vi "Error Q v1_0_1.vi"(0 "Queue name":string="Error", 2 "rendezvous":T1, 3 "error in":errorcluster, 4 "Error Log File":path) -> (10 "error out":errorcluster)   [LabVIEW 2015]
doc: "Error Q v1_0_0.vi\n\nTest Error Control:\n\nProcesses errors and logs them for the Test application.\nthis vi processes any errors that get sent to it. It will build a text file at the location of the file path you provide. It must be either started before your statemachine if ran in the same block diagram. (note in this case it must be ran indepedently from the rest of the state machine. if you wire up the error out indicator it will stop the state machine from running.) The other option is to launch it through vi server or system executive.vi. \n\n\nafter it is started --> send the following command to the Error queue. \"open?True\" or \"open?False\". open tells this vi to put an open statement on the error file. if True is passed to it it will append new entries to the existing file. False tells it to make a new file and delete any existing file. \n\nAt the end of your program --> send the followiing command to the Error queue... \"close\".\nthis will place a close statement in the error file and stop this vi.\n\n\n\nDeveloped by:\n J. Daren Suntych\nNational Analytics 2002\n970-397-0764"
panel:
  in  "Tree":string(tree)
  # "<-  path, including name, for the log file."
  # "<-  rendevouz used to coordinate activities between\n     this VI and the application."
  # "To Avoid creating duplicate Error codes.  Use Ranges of 5000 - 9999 for custom e\ncode development"
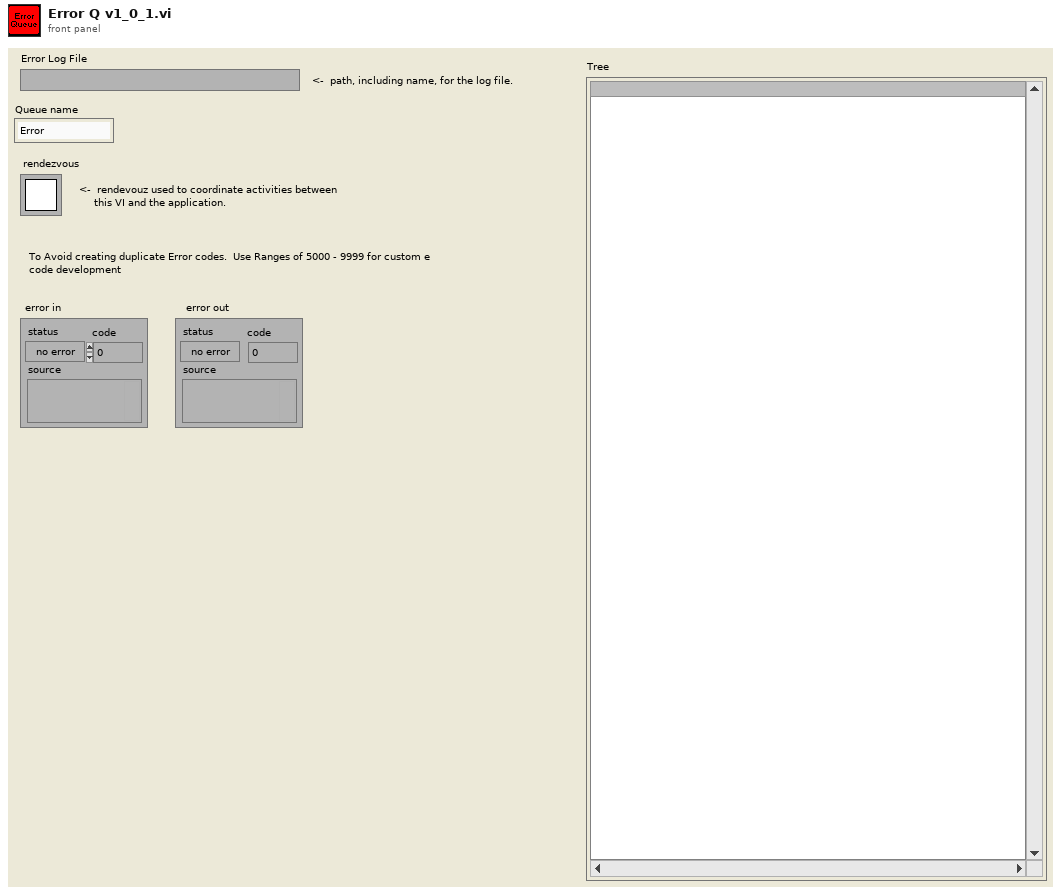
[diagram p1: front panel]
types:
  T1 = typedef "Rendezvous RefNum" = refnum<k1>
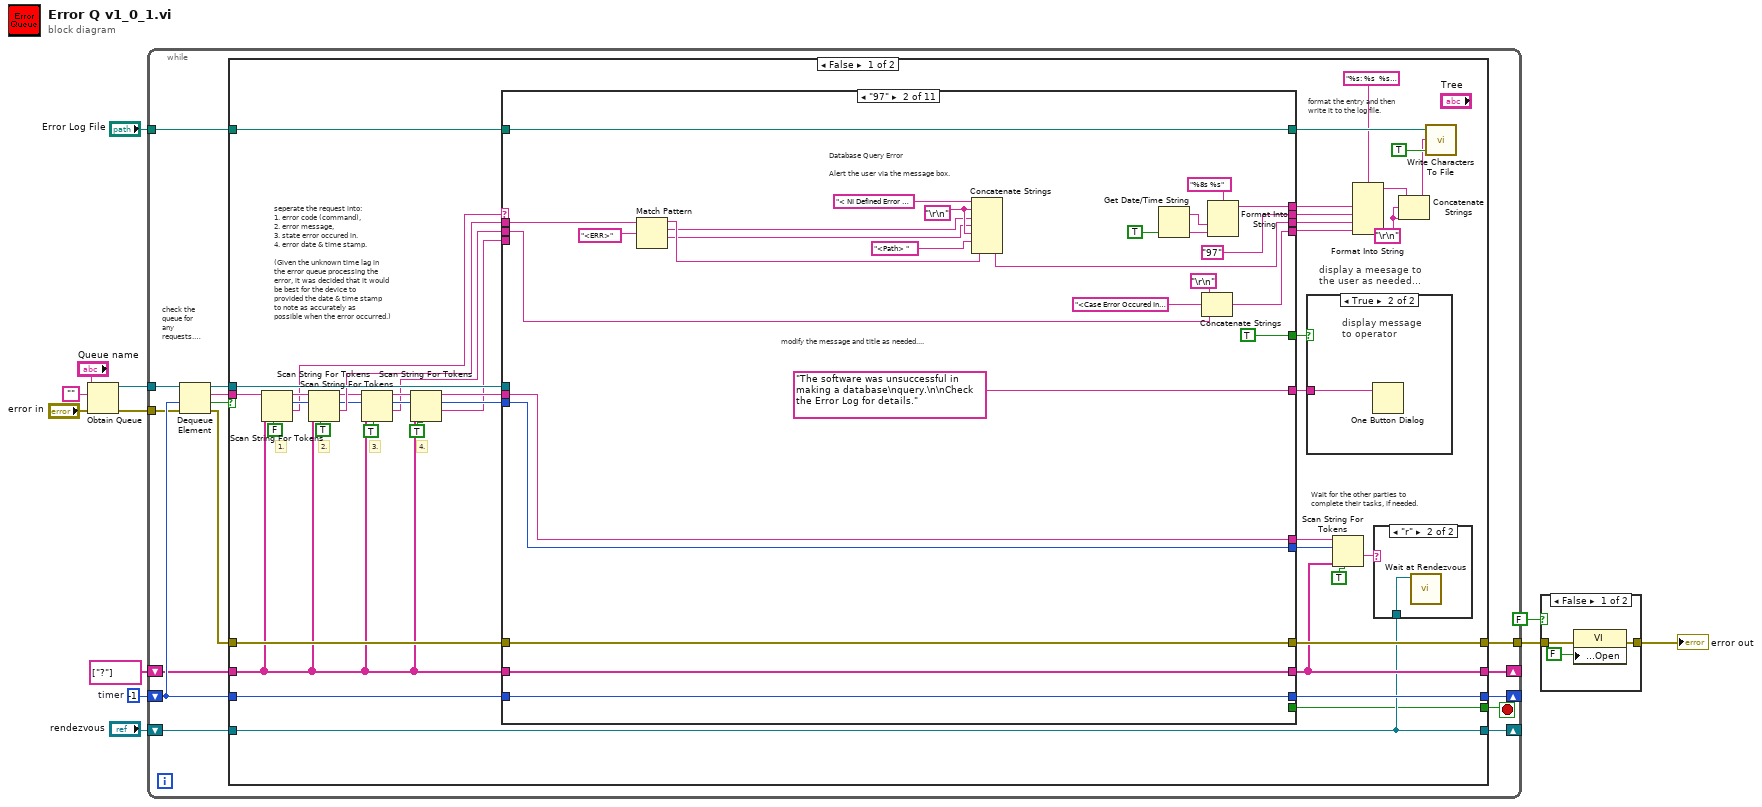
[diagram p0: block diagram]
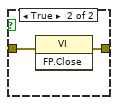
[diagram p2: hidden frame]
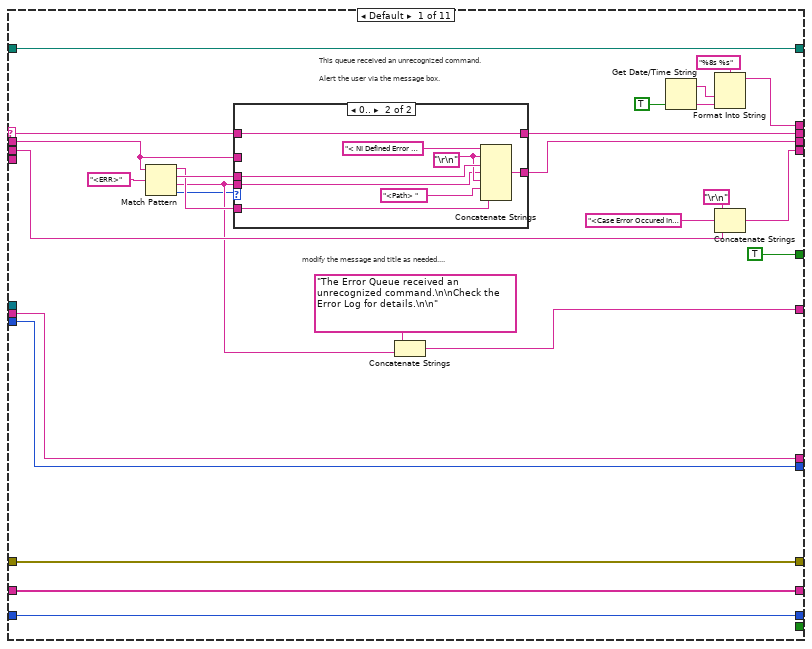
[diagram p5: hidden frame]
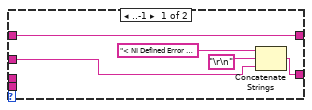
[diagram p6: hidden frame]
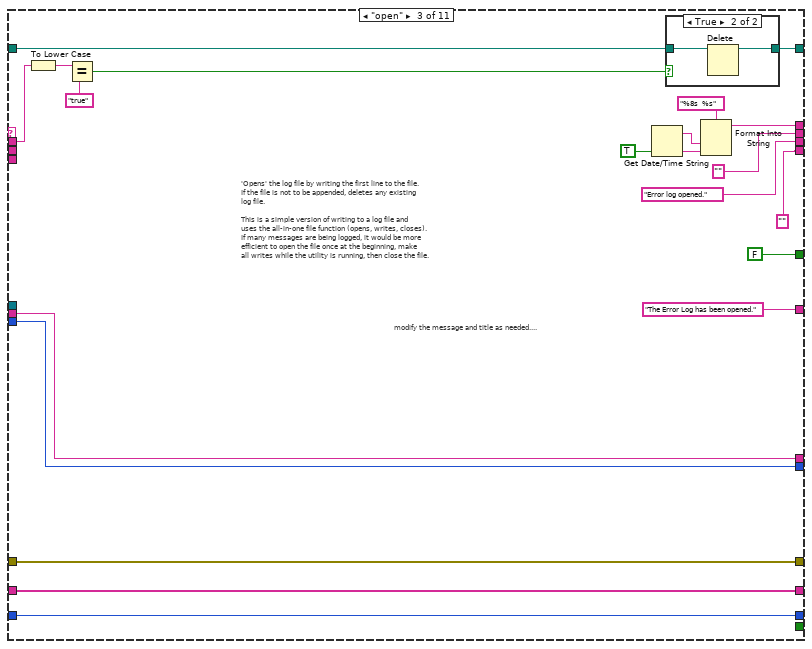
[diagram p7: hidden frame]
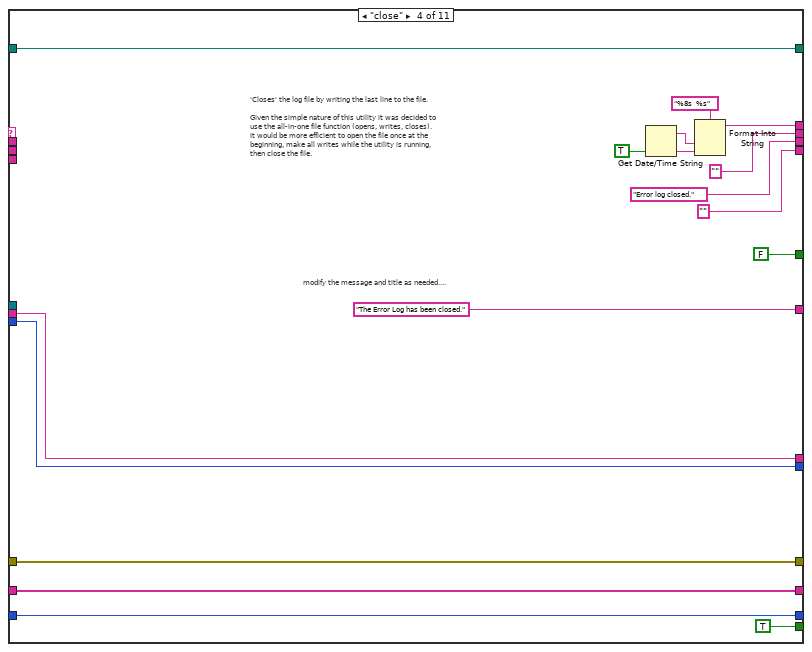
[diagram p9: hidden frame]
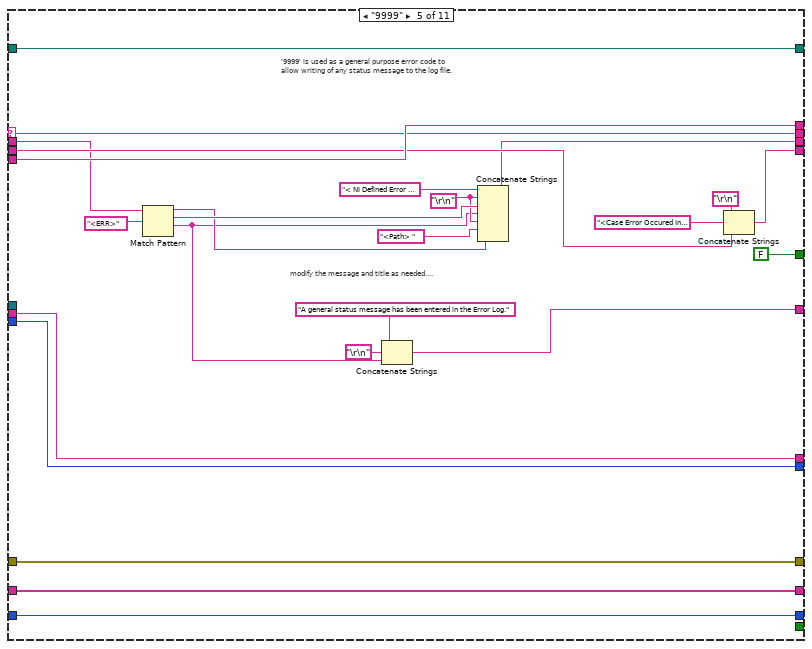
[diagram p10: hidden frame]
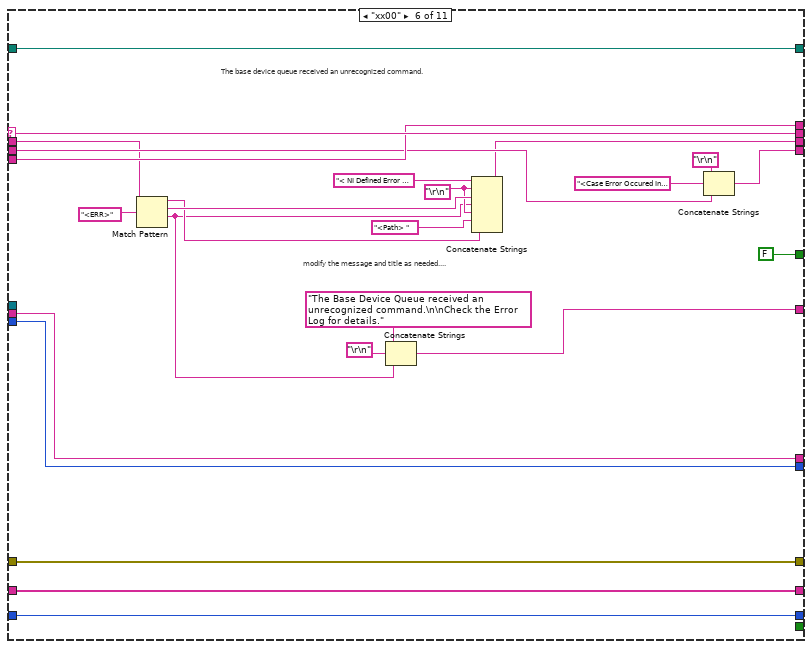
[diagram p11: hidden frame]
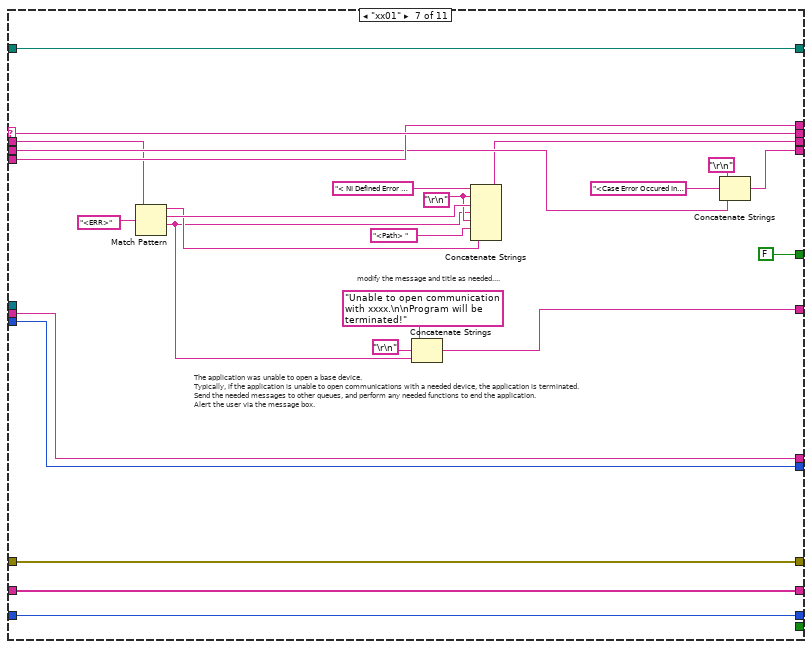
[diagram p12: hidden frame]
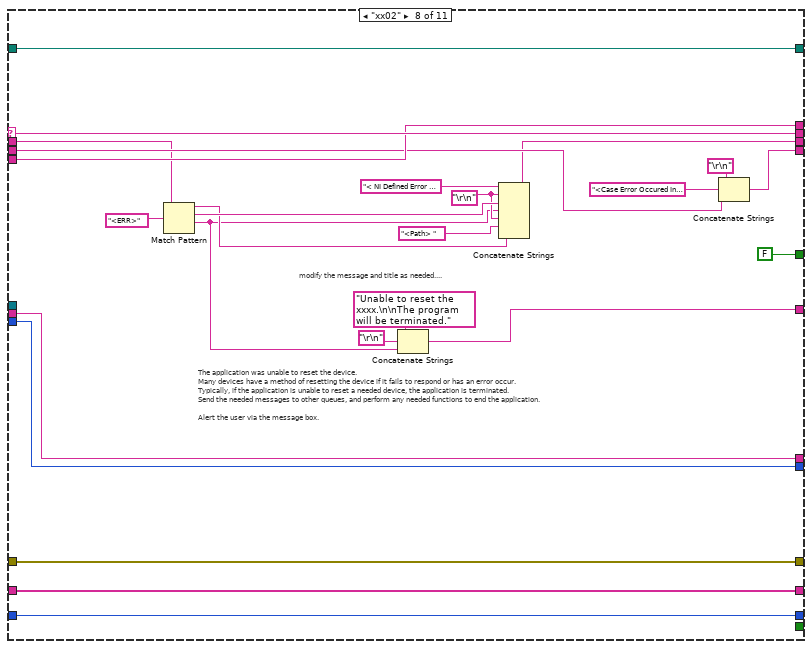
[diagram p13: hidden frame]
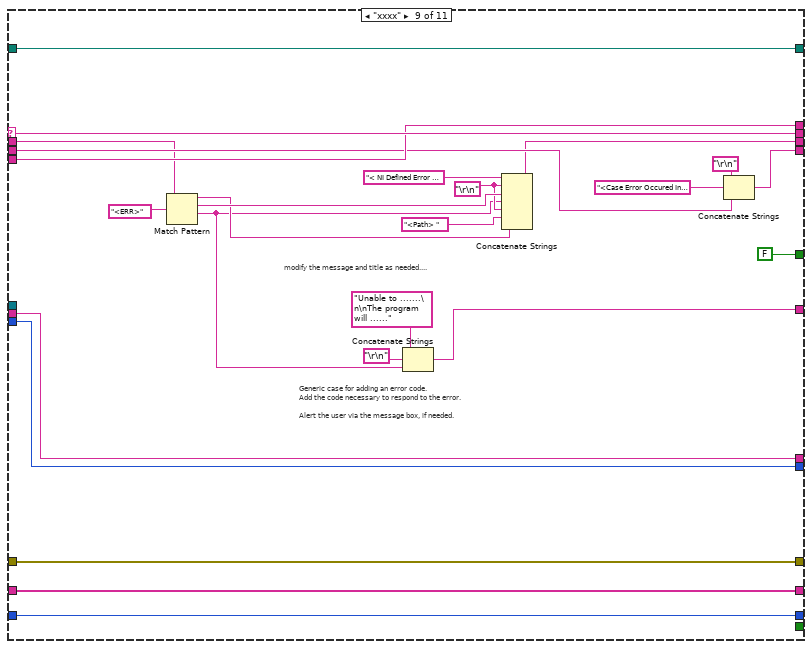
[diagram p14: hidden frame]
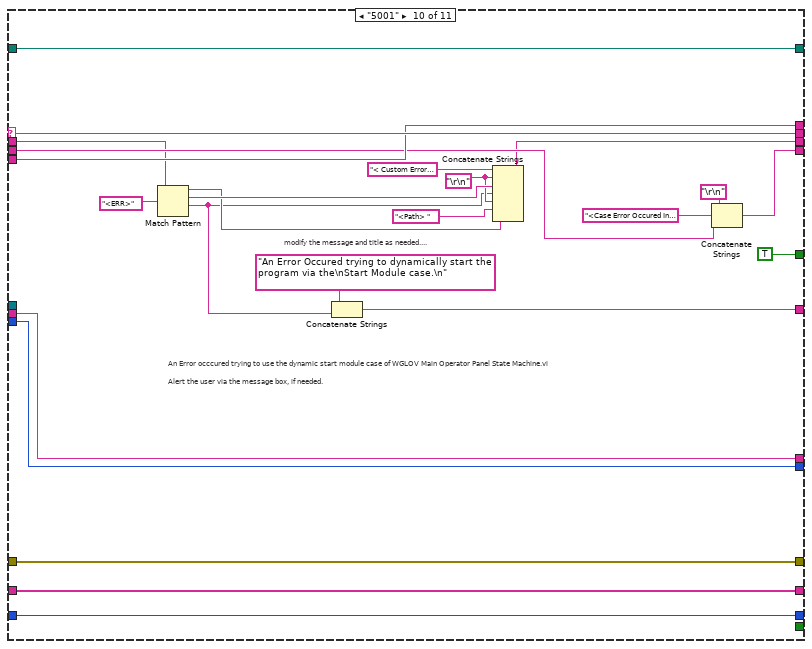
[diagram p15: hidden frame]
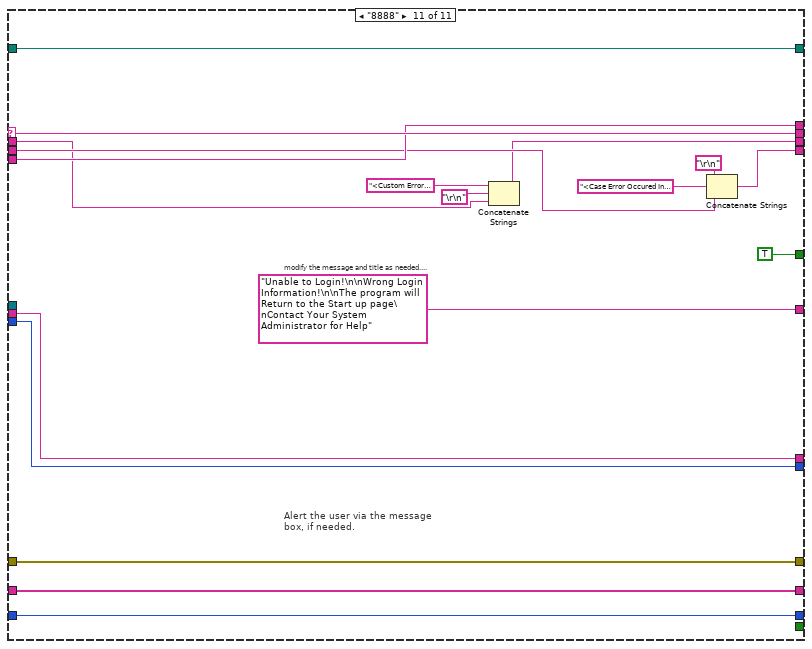
[diagram p16: hidden frame]
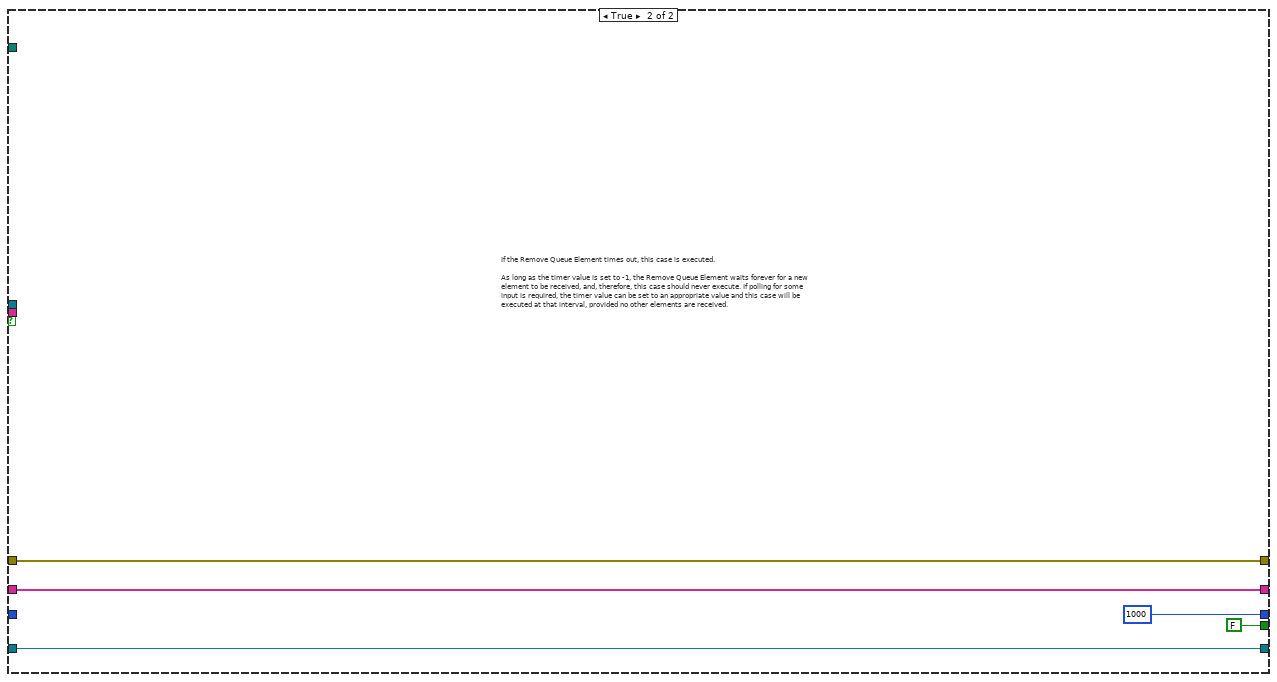
[diagram p17: hidden frame]
diagram:
  w12 = -1  # timer
  n1 = Obtain Queue(name (unnamed)="Queue name", element data type="", error in (no error)="error in") -> (queue out=w7:refnum<queue>, error out=w6:errorcluster)  [unwired: 2 in, 1 out]
  n2 = while {
    shift-left: "rendezvous" -> [w17]
    shift-right: [w16] -> _
    tunnel: "Error Log File" -> [w18]
    shift-left: string[] ["?"] ("Tokens") -> [w21]
    shift-right: [w20] -> _
    tunnel: w7 -> [w26]
    shift-left: w12 -> [w27]
    shift-right: [w22] -> _
    tunnel: [w19] -> w2
    tunnel: w6 -> [w13]
    stop <- w14 stop-if-true
    # "check the \nqueue for\nany \nrequests....."
    n3 = Dequeue Element(queue=w26, timeout in ms (-1)=w27, error in (no error)=w13) -> (queue out=w25:refnum<queue>, element=w24:string, timed out?=w23:bool, error out=w15:errorcluster)
    n4 = case shown="False" w23 {
      tunnel: [w64 w352] -> w19
      tunnel: w27 -> [w70 _]
      tunnel: w25 -> [w69 _]
      tunnel: w24 -> [w66 _]
      tunnel: w15 -> [w68 w352]
      tunnel: [w65 1000 ("timer")] -> w22
      tunnel: w21 -> [w28 w351]
      tunnel: [w48 w351] -> w20
      tunnel: w18 -> [w62 _]
      tunnel: w17 -> [w43 w350]
      tunnel: [w43 w350] -> w16
      tunnel: [w40 FALSE] -> w14
      frame False {
        w30 = "\r\n"
        # "3."
        # "4."
        # "2."
        # "1."
        # "format the entry and then\nwrite it to the log file."
        # "display a meesage to\nthe user as needed..."
        # "seperate the request into:\n1. error code (command),\n2. error message,\n3. state error occured in.\n4. error date & time stamp.\n\n(Given the unknown time lag in\nthe error queue processing the\nerror, it was decided that it would\nbe best for the device to\nprovided the date & time stamp\nto note as accurately as \npossible when the error occurred.)"
        # "Wait for the other parties to\ncomplete their tasks, if needed."
        n5 = Scan String For Tokens(4:FALSE ("use cached delim/oper data? (F)"), 6:w28, 9:w66) -> (1:w41:string, 2:w55:i32, 3:w54:string)  [unwired: 1 in, 3 out]
        n6 = Scan String For Tokens(4:TRUE ("use cached delim/oper data? (F)"), 6:w28, 8:w55, 9:w54) -> (1:w42:string, 2:w37:i32, 3:w39:string)  [unwired: 3 out]
        n7 = Scan String For Tokens(4:TRUE ("use cached delim/oper data? (F)"), 6:w28, 8:w37, 9:w39) -> (1:w35:string, 2:w36:i32, 3:w38:string)  [unwired: 3 out]
        n8 = Scan String For Tokens(4:TRUE ("use cached delim/oper data? (F)"), 6:w28, 8:w36, 9:w38) -> (1:w51:string, 2:w52:i32, 3:w53:string)  [unwired: 3 out]
        n9 = case shown="\"97\"" w41 {
          selector: w41 -> [w76 _ _ _ w199 w227 w253 w277 w302 w326 w344]
          tunnel: [w97 w137 w158 w178 w203 w229 w254 w279 w304 w328 w346] -> w64
          tunnel: w68 -> [w97 w137 w158 w178 w203 w229 w254 w279 w304 w328 w346]
          tunnel: w70 -> [w98 w138 w159 w179 w204 w230 w255 w280 w305 w329 w347]
          tunnel: w69 -> [_ _ _ _ _ _ _ _ _ _ _]
          tunnel: w28 -> [w99 w139 w160 w180 w205 w225 w251 w275 w300 w324 w342]
          tunnel: w52 -> [w89 w129 w145 w166 w197 w222 w248 w272 w297 w321 w339]
          tunnel: [w98 w138 w159 w179 w204 w230 w255 w280 w305 w329 w347] -> w65
          tunnel: [w99 w139 w160 w180 w205 w225 w251 w275 w300 w324 w342] -> w48
          tunnel: w53 -> [w85 w122 w146 w167 w198 w223 w249 w273 w298 w322 w340]
          tunnel: [w91 w131 w157 w177 w202 w228 w247 w278 w303 w327 w345] -> w61
          tunnel: w62 -> [w91 w131 w156 w177 w202 w228 w247 w278 w303 w327 w345]
          tunnel: [w92 w132 w151 w172 w200 w226 w252 w276 w301 w325 w343] -> w60
          tunnel: [w75 "97" "" "" w199 w227 w253 w277 w302 w326 w344] -> w59
          tunnel: [w77 w113 "Error log opened." "Error log closed." w185 w210 w235 w260 w285 w308 w332] -> w58
          tunnel: w42 -> [w73 w114 w144 _ w186 w211 w236 w262 w286 w307 w331]
          tunnel: w51 -> [_ _ _ _ w200 w226 w252 w276 w301 w325 w343]
          tunnel: [w87 "The software was unsuccessful in making a database\nquery.\n\nCheck the Error Log for details." "The Error Log has been opened." "The Error Log has been closed." w182 w207 w232 w257 w281 w320 "Unable to Login!\n\nWrong Login Information!\n\nThe program will Return to the Start up page\nContact Your System Administrator for Help"] -> w50
          tunnel: [TRUE TRUE FALSE FALSE FALSE FALSE FALSE FALSE FALSE TRUE TRUE] -> w49
          tunnel: [w85 w122 w146 w167 w198 w223 w249 w273 w298 w322 w340] -> w45
          tunnel: [w89 w129 w145 w166 w197 w222 w248 w272 w297 w321 w339] -> w44
          tunnel: [_ _ _ TRUE _ _ _ _ _ _ _] -> w40
          tunnel: w35 -> [w82 w123 _ _ w193 w218 w243 w268 w293 w315 w335]
          tunnel: [w86 w124 "" "" w194 w219 w244 w269 w294 w316 w336] -> w33
          frame Default {
            # "modify the message and title as needed...."
            # "This queue received an unrecognized command.\n\nAlert the user via the message box."
            n10 = Match Pattern(string=w73, regular expression="<ERR>") -> (before substring=w79:string, match substring=w80:string, after substring=w78:string, offset past match=w74:i32)  [unwired: 1 out]
            n11 = case shown="0.." w74 {
              tunnel: w80 -> [_ w111]
              tunnel: w79 -> [_ w108]
              tunnel: w78 -> [_ w107]
              tunnel: [w103 w106] -> w77
              tunnel: w76 -> [w102 w105]
              tunnel: [w102 w105] -> w75
              tunnel: w73 -> [w101 _]
              frame ..-1 {
                n12 = Concatenate Strings("< NI Defined Error > ", "\r\n", w101) -> (w103:string)
              }
              frame 0.. {
                w110 = "\r\n"
                n13 = Concatenate Strings("< NI Defined Error > ", w110, w111, w107, w110, "<Path> ", w108) -> (w106:string)
              }
            }
            n14 = Concatenate Strings("The Error Queue received an unrecognized command.\n\nCheck the Error Log for details.\n\n", w78) -> (w87:string)
            n15 = Get Date/Time String(want seconds? (F)=TRUE) -> (date string=w95:string, time string=w94:string)  [unwired: 2 out]
            n16 = Format Into String(format string="%8s %s", w95, w94) -> (resulting string=w92:string)  [unwired: 2 in, 1 out]
            n17 = Concatenate Strings("\r\n", "<Case Error Occured In> ", w82) -> (w86:string)
          }
          frame "97" {
            w119 = "\r\n"
            # "modify the message and title as needed...."
            # "Database Query Error\n\nAlert the user via the message box."
            n18 = Match Pattern(string=w114, regular expression="<ERR>") -> (before substring=w121:string, match substring=w117:string, after substring=w118:string)  [unwired: 2 out]
            n19 = Concatenate Strings("< NI Defined Error > ", w119, w117, w118, w119, "<Path> ", w121) -> (w113:string)
            n20 = Get Date/Time String(want seconds? (F)=TRUE) -> (date string=w135:string, time string=w134:string)  [unwired: 2 out]
            n21 = Concatenate Strings("\r\n", "<Case Error Occured In> ", w123) -> (w124:string)
            n22 = Format Into String(format string="%8s %s", w135, w134) -> (resulting string=w132:string)  [unwired: 2 in, 1 out]
          }
          frame "open" {
            # "modify the message and title as needed...."
            # "'Opens' the log file by writing the first line to the file.\nIf the file is not to be appended, deletes any existing\nlog file.\n\nThis is a simple version of writing to a log file and\nuses the all-in-one file function (opens, writes, closes).\nIf many messages are being logged, it would be more\nefficient to open the file once at the beginning, make\nall writes while the utility is running, then close the file."
            n23 = To Lower Case(string=w144) -> (all lower case string=w142:string)
            n24 = Equal?(x=w142, y="true") -> (x = y?=w141:bool)
            n25 = Get Date/Time String(want seconds? (F)=TRUE) -> (date string=w154:string, time string=w153:string)  [unwired: 2 out]
            n26 = case shown="True" w141 {
              tunnel: w156 -> [w161 w163]
              tunnel: [w161 w162] -> w157
              frame False {
              }
              frame True {
                n27 = Delete(path (use dialog)=w163) -> (deleted path=w162:path)  [unwired: 1 in, 5 out]
              }
            }
            n28 = Format Into String(format string="%8s  %s", w154, w153) -> (resulting string=w151:string)  [unwired: 2 in, 1 out]
          }
          frame "close" {
            # "modify the message and title as needed...."
            # "'Closes' the log file by writing the last line to the file.\n\nGiven the simple nature of this utility it was decided to\nuse the all-in-one file function (opens, writes, closes).\nIt would be more efficient to open the file once at the\nbeginning, make all writes while the utility is running,\nthen close the file."
            n29 = Get Date/Time String(want seconds? (F)=TRUE) -> (date string=w175:string, time string=w174:string)  [unwired: 2 out]
            n30 = Format Into String(format string="%8s  %s", w175, w174) -> (resulting string=w172:string)  [unwired: 2 in, 1 out]
          }
          frame "9999" {
            w190 = "\r\n"
            # "modify the message and title as needed...."
            # "'9999' is used as a general purpose error code to\nallow writing of any status message to the log file."
            n31 = Match Pattern(string=w186, regular expression="<ERR>") -> (before substring=w188:string, match substring=w191:string, after substring=w181:string)  [unwired: 2 out]
            n32 = Concatenate Strings("A general status message has been entered in the Error Log.", "\r\n", w181) -> (w182:string)
            n33 = Concatenate Strings("< NI Defined Error > ", w190, w191, w181, w190, "<Path> ", w188) -> (w185:string)
            n34 = Concatenate Strings("\r\n", "<Case Error Occured In> ", w193) -> (w194:string)
          }
          frame "xx00" {
            w215 = "\r\n"
            # "modify the message and title as needed...."
            # "The base device queue received an unrecognized command."
            n35 = Match Pattern(string=w211, regular expression="<ERR>") -> (before substring=w213:string, match substring=w216:string, after substring=w208:string)  [unwired: 2 out]
            n36 = Concatenate Strings("The Base Device Queue received an unrecognized command.\n\nCheck the Error Log for details.", "\r\n", w208) -> (w207:string)
            n37 = Concatenate Strings("< NI Defined Error > ", w215, w216, w208, w215, "<Path> ", w213) -> (w210:string)
            n38 = Concatenate Strings("\r\n", "<Case Error Occured In> ", w218) -> (w219:string)
          }
          frame "xx01" {
            w239 = "\r\n"
            # "modify the message and title as needed...."
            # "The application was unable to open a base device.\nTypically, if the application is unable to open communications with a needed device, the application is terminated.\nSend the needed messages to other queues, and perform any needed functions to end the application.\nAlert the user via the message box."
            n39 = Match Pattern(string=w236, regular expression="<ERR>") -> (before substring=w237:string, match substring=w240:string, after substring=w231:string)  [unwired: 2 out]
            n40 = Concatenate Strings("Unable to open communication with xxxx.\n\nProgram will be terminated!", "\r\n", w231) -> (w232:string)
            n41 = Concatenate Strings("< NI Defined Error > ", w239, w240, w231, w239, "<Path> ", w237) -> (w235:string)
            n42 = Concatenate Strings("\r\n", "<Case Error Occured In> ", w243) -> (w244:string)
          }
          frame "xx02" {
            w265 = "\r\n"
            # "modify the message and title as needed...."
            # "The application was unable to reset the device.\nMany devices have a method of resetting the device if it fails to respond or has an error occur.\nTypically, if the application is unable to reset a needed device, the application is terminated.\nSend the needed messages to other queues, and perform any needed functions to end the application.\n\nAlert the user via the message box."
            n43 = Match Pattern(string=w262, regular expression="<ERR>") -> (before substring=w263:string, match substring=w266:string, after substring=w256:string)  [unwired: 2 out]
            n44 = Concatenate Strings("Unable to reset the xxxx.\n\nThe program will be terminated.", "\r\n", w256) -> (w257:string)
            n45 = Concatenate Strings("< NI Defined Error > ", w265, w266, w256, w265, "<Path> ", w263) -> (w260:string)
            n46 = Concatenate Strings("\r\n", "<Case Error Occured In> ", w268) -> (w269:string)
          }
          frame "xxxx" {
            w291 = "\r\n"
            # "modify the message and title as needed...."
            # "Generic case for adding an error code.\nAdd the code necessary to respond to the error.\n\nAlert the user via the message box, if needed."
            n47 = Match Pattern(string=w286, regular expression="<ERR>") -> (before substring=w289:string, match substring=w292:string, after substring=w283:string)  [unwired: 2 out]
            n48 = Concatenate Strings("Unable to .......\n\nThe program will ......", "\r\n", w283) -> (w281:string)
            n49 = Concatenate Strings("< NI Defined Error > ", w291, w292, w283, w291, "<Path> ", w289) -> (w285:string)
            n50 = Concatenate Strings("\r\n", "<Case Error Occured In> ", w293) -> (w294:string)
          }
          frame "5001" {
            w312 = "\r\n"
            # "modify the message and title as needed...."
            # "An Error occcured trying to use the dynamic start module case of WGLOV Main Operator Panel State Machine.vi\n\nAlert the user via the message box, if needed."
            n51 = Match Pattern(string=w307, regular expression="<ERR>") -> (before substring=w310:string, match substring=w313:string, after substring=w306:string)  [unwired: 2 out]
            n52 = Concatenate Strings("An Error Occured trying to dynamically start the program via the\nStart Module case.\n", w306) -> (w320:string)
            n53 = Concatenate Strings("< Custom Error > ", w312, w313, w306, w312, "<Path> ", w310) -> (w308:string)
            n54 = Concatenate Strings("\r\n", "<Case Error Occured In> ", w315) -> (w316:string)
          }
          frame "8888" {
            # "modify the message and title as needed...."
            # "Alert the user via the message box, if needed."
            n55 = Concatenate Strings("<Custom Error > ", "\r\n", w331) -> (w332:string)
            n56 = Concatenate Strings("\r\n", "<Case Error Occured In> ", w335) -> (w336:string)
          }
        }
        n57 = case shown="True" w49 {
          tunnel: w50 -> [_ w72]
          frame False {
          }
          frame True {
            # "display message\nto operator"
            n58 = One Button Dialog(message=w72) -> ()  [unwired: 2 out]
          }
        }
        n59 = Scan String For Tokens(4:TRUE ("use cached delim/oper data? (F)"), 6:w48, 8:w44, 9:w45) -> (1:w47:string)  [unwired: 5 out]
        n60 = Format Into String(format string="%s: %s  %s %s", w60, w59, w58, w33) -> (resulting string=w31:string)  [unwired: 2 in, 1 out]
        n61 = case shown="\"r\"" w47 {
          tunnel: w43 -> [_ w71]
          frame Default {
          }
          frame "r" {
            n62 = call <vilib>:"Wait at Rendezvous.vi"("rendezvous"=w71) -> ()  [unwired: 2 in, 5 out]
          }
        }
        n63 = Concatenate Strings(w31, w30, w30) -> (w29:string)
        n64 = call <vilib>:"Write Characters To File.vi"("append to file? (new file:F)"=TRUE, "character string"=w29, "file path (dialog if empty)"=w61) -> ()  [unwired: 3 out]
      }
      frame True {
        # "If the Remove Queue Element times out, this case is executed.\n\nAs long as the timer value is set to -1, the Remove Queue Element waits forever for a new\nelement to be received, and, therefore, this case should never execute. If polling for some\ninput is required, the timer value can be set to an appropriate value and this case will be\nexecuted at that interval, provided no other elements are received."
      }
    }
  }
  n65 = case shown="False" FALSE {
    tunnel: [w354 w357] -> w3
    tunnel: w2 -> [w355 w356]
    frame False {
      n66 = property class="VI"(error in=w355, "Front Panel.Open"=FALSE ("Front Panel Window:Open")) -> (error out=w354:errorcluster)  [unwired: 1 in, 1 out]
    }
    frame True {
      n67 = invoke class="VI" method="FP.Close"(error in=w356) -> (error out=w357:errorcluster)  [unwired: 2 in, 2 out]
    }
  }
  "error out" <- w3
